vi "GetTextInformation.vi"(8 "error in (no error)":errorcluster, 10 "Input":string, 11 "BarCode in":refnum<class "BarCode.lvclass">) -> (0 "error out":errorcluster, 1 "Text":string, 2 "Text Positions":T1[](array[typedef]), 3 "BarCode out":refnum<class "BarCode.lvclass">)   [LabVIEW 2013, in "BarCodes.lvlib" / "BarCode.lvclass"]
doc: "Returns an array of clusters describing how text will be sized and positioned and the actual text to place below the bar code. The Start Index is the index in the returned string that each text info entry refers to. The length is the number of characters in the returned string that each text info entry refers to. The Text Rectangle is the rectangle to draw text in. The Clearing Rectangle is the rectangle to paint with the barcode's light color to make the text clear and visible. The font information is passed into the text writing function."
uses:
  BarCode.lvclass
  TextPosition.ctl
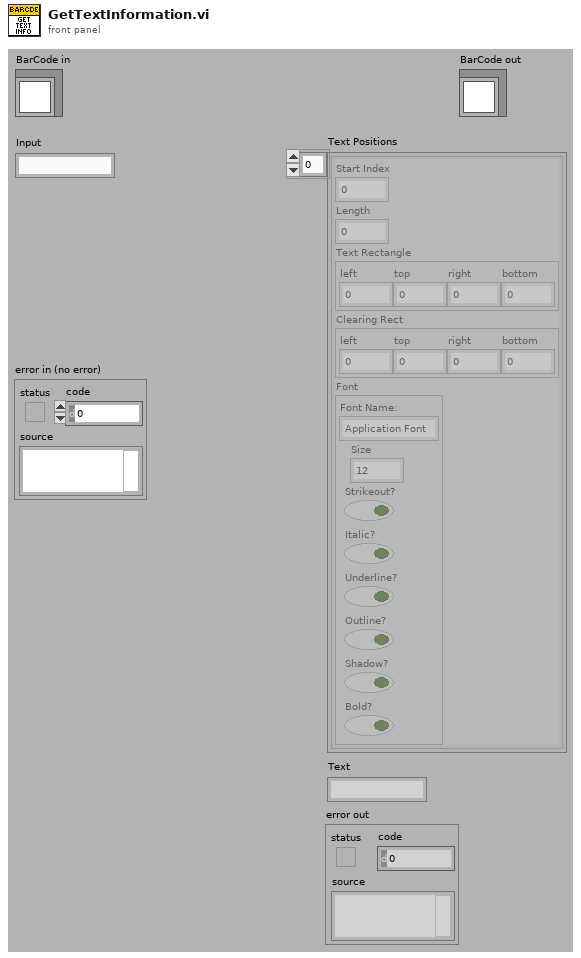
[diagram p1: front panel]
types:
  T1 = typedef "BarCodes.lvlib/BarCode.lvclass/TextPosition.ctl" = cluster{"Start Index":u8, "Length":u8, "Text Rectangle":cluster{"left":i16, "top":i16, "right":i16, "bottom":i16}, "Clearing Rect":cluster{"left":i16, "top":i16, "right":i16, "bottom":i16}, "Font":cluster{"Font Name:":string, "Size":i16, "Strikeout?":bool, "Italic?":bool, "Underline?":bool, "Outline?":bool, "Shadow?":bool, "Bold?":bool}}
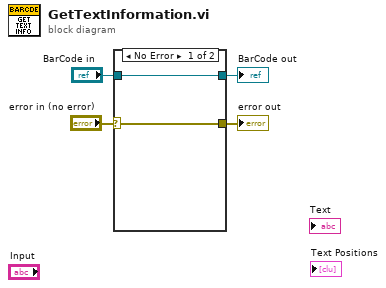
[diagram p0: block diagram]
diagram:
  n1 = case shown="No Error" "error in (no error)" {
    selector: "error in (no error)" -> [w5 w8]
    tunnel: [w5 w8] -> w3
    tunnel: [w6 w7] -> w1
    tunnel: "BarCode in" -> [w6 w7]
    frame No Error {
    }
    frame Error {
    }
  }
  "error out" <- w3
  "BarCode out" <- w1
